vi "LVClass_ModalCoef Write ModalCoef ptr create.vi"(8 "error in (no error)":errorcluster, 10 "Enum":T1, 11 "ModalCoef in":refnum<class "ModalCoef.lvclass">) -> (0 "error out":errorcluster, 3 "ModalCoef out":refnum<class "ModalCoef.lvclass">)   [LabVIEW 2020, in "ModalCoef.lvclass"]
uses:
  ModalCoef.lvclass
  Handle creation.ctl
  ModalCoef.lvclass/ModalCoef.ctl
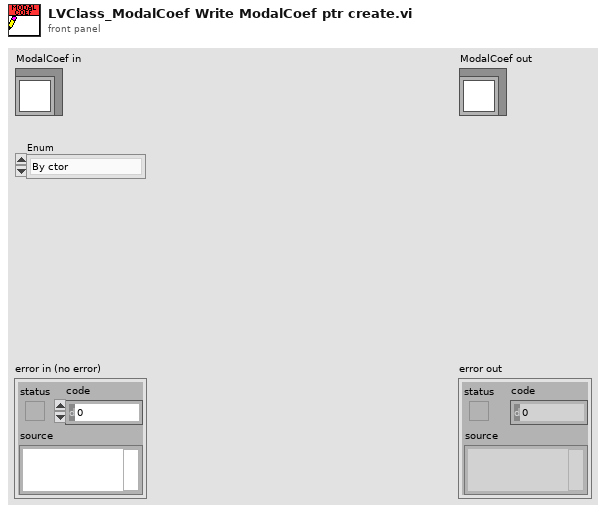
[diagram p1: front panel]
types:
  T1 = typedef "Handle creation.ctl" = enum16{"By ctor", "By write function"}
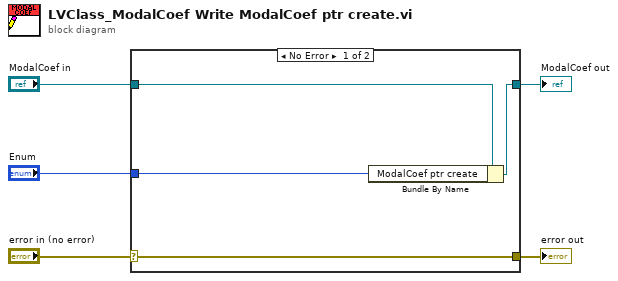
[diagram p0: block diagram]
diagram:
  n1 = case shown="No Error" "error in (no error)" {
    selector: "error in (no error)" -> [w9 w10]
    tunnel: [w9 w10] -> w4
    tunnel: [w7 w11] -> w2
    tunnel: "ModalCoef in" -> [w8 w11]
    tunnel: "Enum" -> [w6 _]
    frame No Error {
      n2 = Bundle By Name(cluster=w8, "ModalCoef ptr create"=w6) -> (w7:refnum<class "ModalCoef.lvclass">)
    }
    frame Error {
    }
  }
  "error out" <- w4
  "ModalCoef out" <- w2
